vi "_LoadPeakSearchParameters.vi"(4 "error in (no error)":errorcluster, 7 "Path":path) -> (0 "error out":errorcluster, 2 "SearchParameters":string, 3 "PeakSearchParameters":dbl[](array[numeric]))   [LabVIEW 2015]
uses:
  Type/_Log Command.ctl
  <vilib>/xml/Load XML File.vi
  <vilib>/xml/Close Reference(Node).vi
  <vilib>/xml/NI_XML.lvlib
  <resource>/objmgr/DOMUserDefRef.rc
panel:
  # "SpectraThresholdPercent"
  # "SpectraThresholdCps"
  # "SpectraLabelPrecision"
  # "SpectraCentroidHeight"
  # "SpectraCentroidWidth"
  # "SpectraNoiseThreshold"
  # "MinimumSlopeToUsePeakMax"
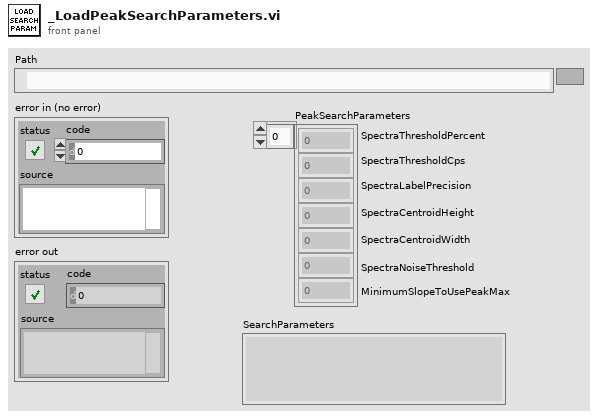
[diagram p1: front panel]
types:
  T1 = typedef "_Log Command.ctl" = enum16{"No Command", "Open", "Read", "Write", "Close", "Check Size"}
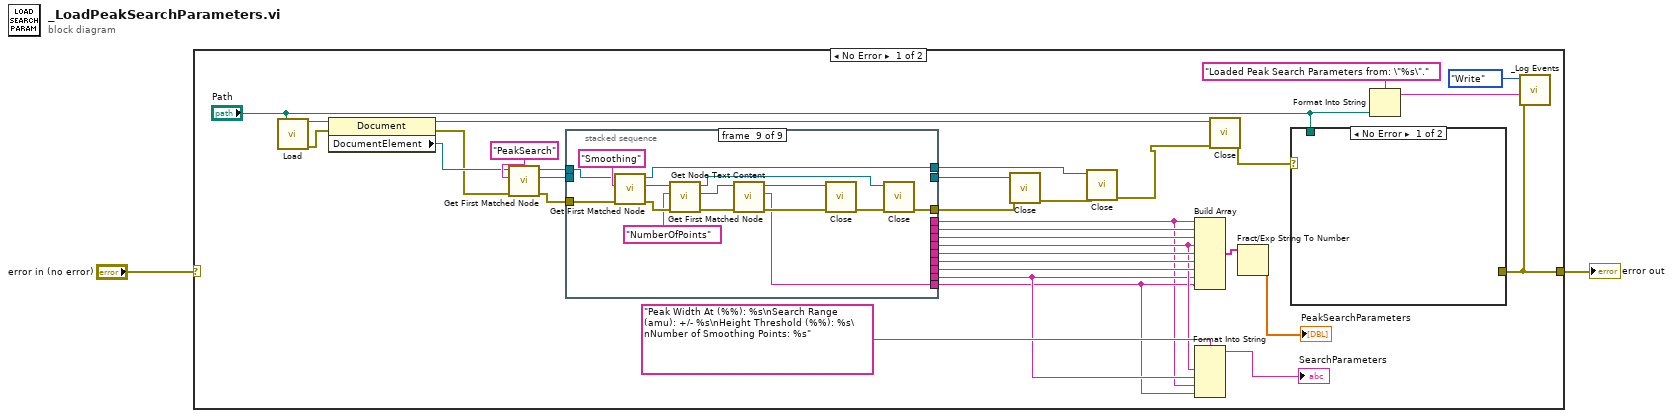
[diagram p0: block diagram]
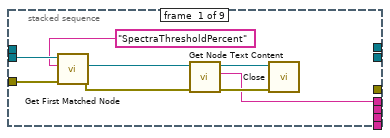
[diagram p2: hidden frame]
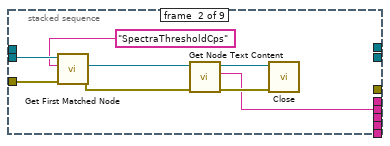
[diagram p3: hidden frame]
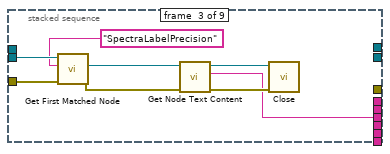
[diagram p4: hidden frame]
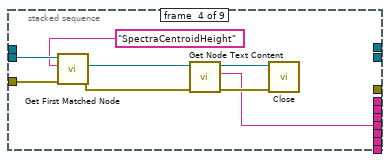
[diagram p5: hidden frame]
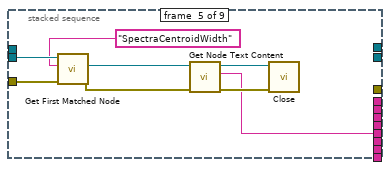
[diagram p6: hidden frame]
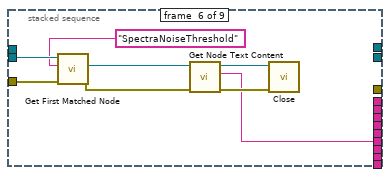
[diagram p7: hidden frame]
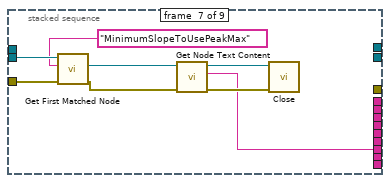
[diagram p8: hidden frame]
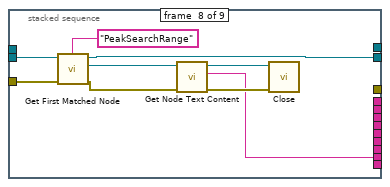
[diagram p9: hidden frame]
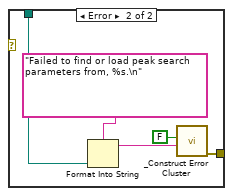
[diagram p10: hidden frame]
diagram:
  n1 = case shown="No Error" "error in (no error)" {
    selector: "error in (no error)" -> [_ w121]
    tunnel: [w27 w121] -> w2
    frame No Error {
      n2 = call-poly <vilib>:"Load.vi"("path to XML document"="Path") -> ("DOM document out"=w35:refnum<k20>, "error out"=w34:errorcluster)  [unwired: 12 in, 1 out]
      n3 = property on="Property Node" class="Document"(reference=w35, error in=w34) -> (reference out=w33:refnum<k20>, error out=w13:errorcluster, "DocumentElement"=w14:refnum<k20>)
      n4 = call <vilib>:"Get First Matched Node.vi"("error in (no error)"=w13, "XPath expression"="PeakSearch", "node in"=w14) -> ("error out"=w15:errorcluster, "node result"=w16:refnum<k20>, "node out"=w5:refnum<k20>)  [unwired: 6 in]
      n5 = stacked-sequence {
        tunnel: w16 -> [w43 w51 w59 w67 w75 w83 w91 w100 _]
        tunnel: w15 -> [w42 w50 w58 w66 w74 w82 w90 w99 w115]
        tunnel: [_ _ _ _ _ _ _ w92 _] -> w26
        tunnel: [_ _ _ _ _ _ _ _ w103] -> w25
        tunnel: [_ w44 _ _ _ _ _ _ _] -> w8
        tunnel: [_ _ w52 _ _ _ _ _ _] -> w18
        tunnel: [_ _ _ w60 _ _ _ _ _] -> w9
        tunnel: [_ _ _ _ w68 _ _ _ _] -> w10
        tunnel: [_ _ _ _ _ w76 _ _ _] -> w19
        tunnel: [_ _ _ _ _ _ w84 _ _] -> w24
        tunnel: [w36 _ _ _ _ _ _ _ _] -> w3
        tunnel: [_ _ _ _ _ _ _ w93 _] -> w7
        tunnel: [_ _ _ _ _ _ _ _ w111] -> w6
        tunnel: w5 -> [_ _ _ _ _ _ _ _ w107]
        tunnel: [_ _ _ _ _ _ _ _ w106] -> w4
        frame #0 {
          n6 = call <vilib>:"Get First Matched Node.vi"("error in (no error)"=w42, "XPath expression"="SpectraThresholdPercent", "node in"=w43) -> ("error out"=w37:errorcluster, "node result"=w40:refnum<k20>)  [unwired: 6 in, 1 out]
          n7 = call <vilib>:"Get Node Text Content.vi"("error in (no error)"=w37, "node in"=w40) -> ("error out"=w38:errorcluster, "node text"=w36:string, "node out"=w39:refnum<k20>)  [unwired: 7 in]
          n8 = call-poly <vilib>:"Close.vi"("error in (no error)"=w38, "node"=w39) -> ()  [unwired: 7 in, 1 out]
        }
        frame #1 {
          n9 = call <vilib>:"Get First Matched Node.vi"("error in (no error)"=w50, "XPath expression"="SpectraThresholdCps", "node in"=w51) -> ("error out"=w45:errorcluster, "node result"=w48:refnum<k20>)  [unwired: 6 in, 1 out]
          n10 = call <vilib>:"Get Node Text Content.vi"("error in (no error)"=w45, "node in"=w48) -> ("error out"=w46:errorcluster, "node text"=w44:string, "node out"=w47:refnum<k20>)  [unwired: 7 in]
          n11 = call-poly <vilib>:"Close.vi"("error in (no error)"=w46, "node"=w47) -> ()  [unwired: 7 in, 1 out]
        }
        frame #2 {
          n12 = call <vilib>:"Get First Matched Node.vi"("error in (no error)"=w58, "XPath expression"="SpectraLabelPrecision", "node in"=w59) -> ("error out"=w53:errorcluster, "node result"=w56:refnum<k20>)  [unwired: 6 in, 1 out]
          n13 = call <vilib>:"Get Node Text Content.vi"("error in (no error)"=w53, "node in"=w56) -> ("error out"=w54:errorcluster, "node text"=w52:string, "node out"=w55:refnum<k20>)  [unwired: 7 in]
          n14 = call-poly <vilib>:"Close.vi"("error in (no error)"=w54, "node"=w55) -> ()  [unwired: 7 in, 1 out]
        }
        frame #3 {
          n15 = call <vilib>:"Get First Matched Node.vi"("error in (no error)"=w66, "XPath expression"="SpectraCentroidHeight", "node in"=w67) -> ("error out"=w61:errorcluster, "node result"=w64:refnum<k20>)  [unwired: 6 in, 1 out]
          n16 = call <vilib>:"Get Node Text Content.vi"("error in (no error)"=w61, "node in"=w64) -> ("error out"=w62:errorcluster, "node text"=w60:string, "node out"=w63:refnum<k20>)  [unwired: 7 in]
          n17 = call-poly <vilib>:"Close.vi"("error in (no error)"=w62, "node"=w63) -> ()  [unwired: 7 in, 1 out]
        }
        frame #4 {
          n18 = call <vilib>:"Get First Matched Node.vi"("error in (no error)"=w74, "XPath expression"="SpectraCentroidWidth", "node in"=w75) -> ("error out"=w69:errorcluster, "node result"=w72:refnum<k20>)  [unwired: 6 in, 1 out]
          n19 = call <vilib>:"Get Node Text Content.vi"("error in (no error)"=w69, "node in"=w72) -> ("error out"=w70:errorcluster, "node text"=w68:string, "node out"=w71:refnum<k20>)  [unwired: 7 in]
          n20 = call-poly <vilib>:"Close.vi"("error in (no error)"=w70, "node"=w71) -> ()  [unwired: 7 in, 1 out]
        }
        frame #5 {
          n21 = call <vilib>:"Get First Matched Node.vi"("error in (no error)"=w82, "XPath expression"="SpectraNoiseThreshold", "node in"=w83) -> ("error out"=w77:errorcluster, "node result"=w80:refnum<k20>)  [unwired: 6 in, 1 out]
          n22 = call <vilib>:"Get Node Text Content.vi"("error in (no error)"=w77, "node in"=w80) -> ("error out"=w78:errorcluster, "node text"=w76:string, "node out"=w79:refnum<k20>)  [unwired: 7 in]
          n23 = call-poly <vilib>:"Close.vi"("error in (no error)"=w78, "node"=w79) -> ()  [unwired: 7 in, 1 out]
        }
        frame #6 {
          n24 = call <vilib>:"Get First Matched Node.vi"("error in (no error)"=w90, "XPath expression"="MinimumSlopeToUsePeakMax", "node in"=w91) -> ("error out"=w87:errorcluster, "node result"=w88:refnum<k20>)  [unwired: 6 in, 1 out]
          n25 = call <vilib>:"Get Node Text Content.vi"("error in (no error)"=w87, "node in"=w88) -> ("error out"=w85:errorcluster, "node text"=w84:string, "node out"=w86:refnum<k20>)  [unwired: 7 in]
          n26 = call-poly <vilib>:"Close.vi"("error in (no error)"=w85, "node"=w86) -> ()  [unwired: 7 in, 1 out]
        }
        frame #7 {
          n27 = call <vilib>:"Get First Matched Node.vi"("error in (no error)"=w99, "XPath expression"="PeakSearchRange", "node in"=w100) -> ("error out"=w96:errorcluster, "node result"=w97:refnum<k20>, "node out"=w92:refnum<k20>)  [unwired: 6 in]
          n28 = call <vilib>:"Get Node Text Content.vi"("error in (no error)"=w96, "node in"=w97) -> ("error out"=w94:errorcluster, "node text"=w93:string, "node out"=w95:refnum<k20>)  [unwired: 7 in]
          n29 = call-poly <vilib>:"Close.vi"("error in (no error)"=w94, "node"=w95) -> ()  [unwired: 7 in, 1 out]
        }
        frame #8 {
          n30 = call <vilib>:"Get First Matched Node.vi"("error in (no error)"=w115, "XPath expression"="Smoothing", "node in"=w107) -> ("error out"=w108:errorcluster, "node result"=w109:refnum<k20>, "node out"=w106:refnum<k20>)  [unwired: 6 in]
          n31 = call <vilib>:"Get First Matched Node.vi"("error in (no error)"=w108, "XPath expression"="NumberOfPoints", "node in"=w109) -> ("error out"=w110:errorcluster, "node result"=w101:refnum<k20>, "node out"=w102:refnum<k20>)  [unwired: 6 in]
          n32 = call <vilib>:"Get Node Text Content.vi"("error in (no error)"=w110, "node in"=w101) -> ("error out"=w112:errorcluster, "node text"=w111:string, "node out"=w113:refnum<k20>)  [unwired: 7 in]
          n33 = call-poly <vilib>:"Close.vi"("error in (no error)"=w112, "node"=w113) -> ("error out"=w104:errorcluster)  [unwired: 7 in]
          n34 = call-poly <vilib>:"Close.vi"("error in (no error)"=w104, "node"=w102) -> ("error out"=w103:errorcluster)  [unwired: 7 in]
        }
      }
      n35 = call-poly <vilib>:"Close.vi"("error in (no error)"=w25, "node"=w26) -> ("error out"=w12:errorcluster)  [unwired: 7 in]
      n36 = call-poly <vilib>:"Close.vi"("error in (no error)"=w12, "node"=w4) -> ("error out"=w11:errorcluster)  [unwired: 7 in]
      n37 = Build Array(w3, w8, w18, w9, w10, w19, w24, w7, w6) -> (w23:string[])
      n38 = Format Into String(format string="Peak Width At (%%): %s\nSearch Range (amu): +/- %s\nHeight Threshold (%%): %s\nNumber of Smoothing Points: %s", w9, w7, w3, w6) -> (resulting string=→"SearchParameters":string)  [unwired: 2 in, 1 out]
      n39 = call-poly <vilib>:"Close.vi"("error in (no error)"=w11, "node"=w33) -> ("error out"=w32:errorcluster)  [unwired: 7 in]
      n40 = Fract/Exp String To Number(string=w23) -> (number=→"PeakSearchParameters":dbl[])  [unwired: 3 in, 1 out]
      n41 = case shown="No Error" w32 {
        tunnel: "Path" -> [_ w118]
        tunnel: [_ w117] -> w27
        frame No Error {
        }
        frame Error {
          n42 = Format Into String(format string="Failed to find or load peak search parameters from, %s.\n", w118) -> (resulting string=w120:string)  [unwired: 2 in, 1 out]
          n43 = call "_Construct Error Cluster.vi"("reason"=w120, "CallingChain? (T)"=FALSE) -> ("error out"=w117:errorcluster)  [unwired: 5 in]
        }
      }
      n44 = Format Into String(format string="Loaded Peak Search Parameters from: \"%s\".", "Path") -> (resulting string=w28:string)  [unwired: 2 in, 1 out]
      n45 = call "_Log Events.vi"("error in (no error)"=w27, "Event"=w28, "Log Command"=_Log_Command."Write" ("File Command")) -> ()  [unwired: 5 in, 2 out]
    }
    frame Error {
    }
  }
  "error out" <- w2
